vi "ReplaceDependency.vi"(8 "error in (no error)":errorcluster, 9 "New dependency":string, 10 "Current dependency":string, 11 "ProjectItem in":refnum<class "ProjectItem.lvclass">) -> (0 "error out":errorcluster, 3 "ProjectItem out":refnum<class "ProjectItem.lvclass">)   [LabVIEW 2019, in "SolutionBuilder.lvlib" / "ProjectItem.lvclass"]
uses:
  ProjectItem.lvclass
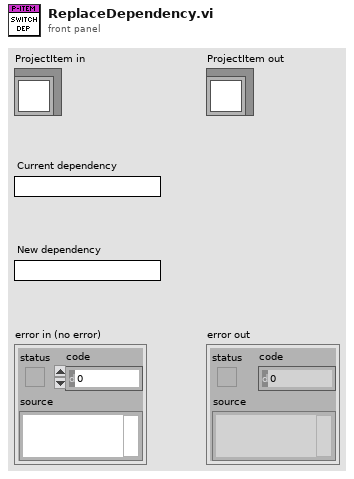
[diagram p1: front panel]
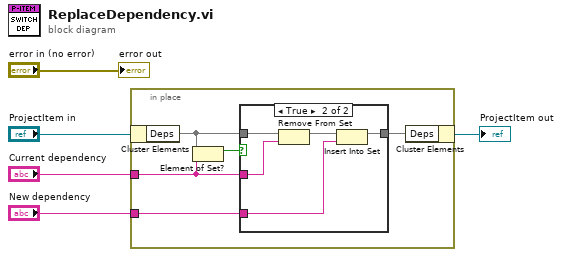
[diagram p0: block diagram]
diagram:
  n1 = in-place {
    in-place-border: "New dependency" -> [w7]
    in-place-border: "Current dependency" -> [w8]
    n2 = in-place-cluster #1("ProjectItem in") -> ("Deps"=w9:set{string})
    n3 = Element of Set?(10:w8, 11:w9) -> (3:w10:bool)
    n4 = case shown="True" w10 {
      tunnel: w9 -> [w11 w16]
      tunnel: w8 -> [_ w15]
      tunnel: w7 -> [_ w13]
      tunnel: [w11 w12] -> w6
      frame False {
      }
      frame True {
        n5 = Remove From Set(10:w15, 11:w16) -> (3:w14:set{string})  [unwired: 1 out]
        n6 = Insert Into Set(10:w13, 11:w14) -> (3:w12:set{string})  [unwired: 1 out]
      }
    }
    n7 = in-place-cluster #1("Deps"=w6) -> (→"ProjectItem out":refnum<class "ProjectItem.lvclass">)
  }
  "error out" <- "error in (no error)"
